vi "Begin.vi"() -> (0 "error out":errorcluster)   [LabVIEW 2013]
doc: "Called before other user functions, this VI is expected to open initial I/O refnums, load in file data, and do all program initialization. Notice that the <B>error out</B> terminal is simply used for data flow. Wiring it to other structures or subVIs ensures that this VI runs first."
uses:
  <vilib>/Rock Robotics/SystemInterfaces/DIO/FPGA_DIOPWMChannel.ctl
  <vilib>/Rock Robotics/WPI/SafetyOutput/WPI_SafetyOutputConfigMenu.ctl
  <vilib>/Rock Robotics/WPI/DriverStation/WPI_DriverStationRobotMode2.ctl
  <vilib>/Rock Robotics/WPI/Joystick/WPI_JoystickDeviceEnum.ctl
  <vilib>/Rock Robotics/SystemInterfaces/DIO/FPGA_DIORelayChannel.ctl
  <vilib>/Rock Robotics/SystemInterfaces/DIO/FPGA_DIOChannel.ctl
  <vilib>/Rock Robotics/SystemInterfaces/Typedef/FPGA_TypedefDigitalModule.ctl
  QueueAction.ctl
  <vilib>/Rock Robotics/WPI/Solenoid/WPI_SolenoidChannel.ctl
  TankDriveAction.ctl
  <vilib>/Rock Robotics/SystemInterfaces/Typedef/FPGA_TypedefSolenoidModule.ctl
  DoubleSolenoidAction.ctl
  RollerAction.ctl
  <vilib>/Rock Robotics/WPI/RobotDrive/WPI_RobotDriveOpen2MotorWithTalon.vi
  Robot Global Data.vi
  OutputErrors.vi
  <vilib>/Rock Robotics/WPI/Solenoid/WPI_SolenoidOpenSingle.vi
  <vilib>/Rock Robotics/WPI/Compressor/WPI_CompressorGetSetRefNum.vi
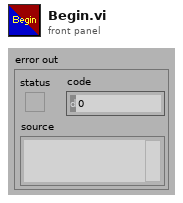
[diagram p1: front panel]
types:
  T1 = typedef "RollerAction.ctl" = enum16{"Init", "Off", "Forward", "Reverse"}
  T2 = typedef "FPGA_DIORelayChannel.ctl" = enum8{"Relay 1", "Relay 2", "Relay 3", "Relay 4", "Relay 5", "Relay 6", "Relay 7", "Relay 8", "Invalid"}
  T3 = typedef "FPGA_TypedefDigitalModule.ctl" = enum16{"Digital Module 1", "Digital Module 2"}
  T4 = typedef "DoubleSolenoidAction.ctl" = enum16{"Init", "Middle", "In", "Out"}
  T5 = typedef "WPI_SolenoidChannel.ctl" = enum8{"Solenoid 1", "Solenoid 2", "Solenoid 3", "Solenoid 4", "Solenoid 5", "Solenoid 6", "Solenoid 7", "Solenoid 8", "Invalid"}
  T6 = typedef "FPGA_TypedefSolenoidModule.ctl" = enum16{"Solenoid Module 1", "Solenoid Module 2"}
  T7 = typedef "QueueAction.ctl" = enum16{"Init", "SetValue", "Disable"}
  T8 = typedef "TankDriveAction.ctl" = enum16{"Init", "LinearDrive", "SetValue", "Disable"}
  T9 = typedef "WPI_JoystickDeviceEnum.ctl" = enum16{"USB 1", "USB 2", "USB 3", "USB 4", "Kinect 1", "Kinect 2"}
  T10 = typedef "FPGA_DIOChannel.ctl" = enum8{"DIO 1", "DIO 2", "DIO 3", "DIO 4", "DIO 5", "DIO 6", "DIO 7", "DIO 8", "DIO 9", "DIO 10", "DIO 11", "DIO 12", "DIO 13", "DIO 14", "Invalid"}
  T11 = typedef "WPI_DriverStationRobotMode2.ctl" = enum16{"Autonomous Disabled", "Autonomous Enabled", "Teleop Disabled", "Teleop Enabled", "Timeout", "Finish", "Test Disabled", "Test Enabled"}
  T12 = typedef "WPI_SafetyOutputConfigMenu.ctl" = enum16{"Enable", "Disable"}
  T13 = typedef "FPGA_DIOPWMChannel.ctl" = enum8{"PWM 1", "PWM 2", "PWM 3", "PWM 4", "PWM 5", "PWM 6", "PWM 7", "PWM 8", "PWM 9", "PWM 10", "Invalid"}
  T14 = typedef "WPI_JoystickDevRef.ctl" = cluster{"Device":T9}
  T15 = typedef "WPI_RobotDriveDevRef.ctl" = cluster{"DevStatus":errorcluster, "Motors[]":T16[], "Square Inputs":bool, "Max Output":dbl, "Isochronous":bool}
  T16 = typedef "WPI_MotorControlDeviceRef.ctl" = cluster{"DeviceStatus":errorcluster, "Type":enum16{"PWM", "CAN"}, "PWM":cluster{"Digital Module":T3, "PWM Channel":T13, "DeadBand":T17}, "CAN":cluster{"Device Number":u8, "Control Mode":T18, "Semaphore":T19, "Max Vout":dbl}, "Invert":bool, "TransformRef":T20, "InvTransformRef":T20}
  T17 = typedef "WPI_PWMDeadband.ctl" = cluster{"Name":string, "maxPositivePwm":i32, "minPositivePwm":i32, "centerPwm":i32, "maxNegativePwm":i32, "minNegativePwm":i32, "angularRange":u16}
  T18 = typedef "WPI_CANJaguar_ControlMode.ctl" = enum8{"Percent VBus", "Current", "Speed", "Position", "Voltage"}
  T19 = typedef "Semaphore RefNum" = refnum<k1>
  T20 = typedef "WPI_PWMTransform_ConPane.ctl" = refnum<vi>
  T21 = typedef "WPI_CompressorDevRef.ctl" = cluster{"DevStatus":errorcluster, "DigitalInputDevRef":T22, "RelayDevRef":T23}
  T22 = typedef "WPI_DigitalInputDevRef.ctl" = cluster{"DevStatus":errorcluster, "DIO Channel":T10, "Digital Module":T3}
  T23 = typedef "WPI_RelayDevRef.ctl" = cluster{"DevStatus":errorcluster, "Relay Channel":T2, "Digital Module":T3, "Relay Direction":T24}
  T24 = typedef "WPI_RelayDirection.ctl" = enum16{"Both directions", "Forward only", "Reverse only"}
  T25 = typedef "WPI_SolenoidDevRef.ctl" = cluster{"DevStatus":errorcluster, "Solenoid Module":T6, "Forward Solenoid Channel":T5, "Reverse Solenoid Channel":T5}
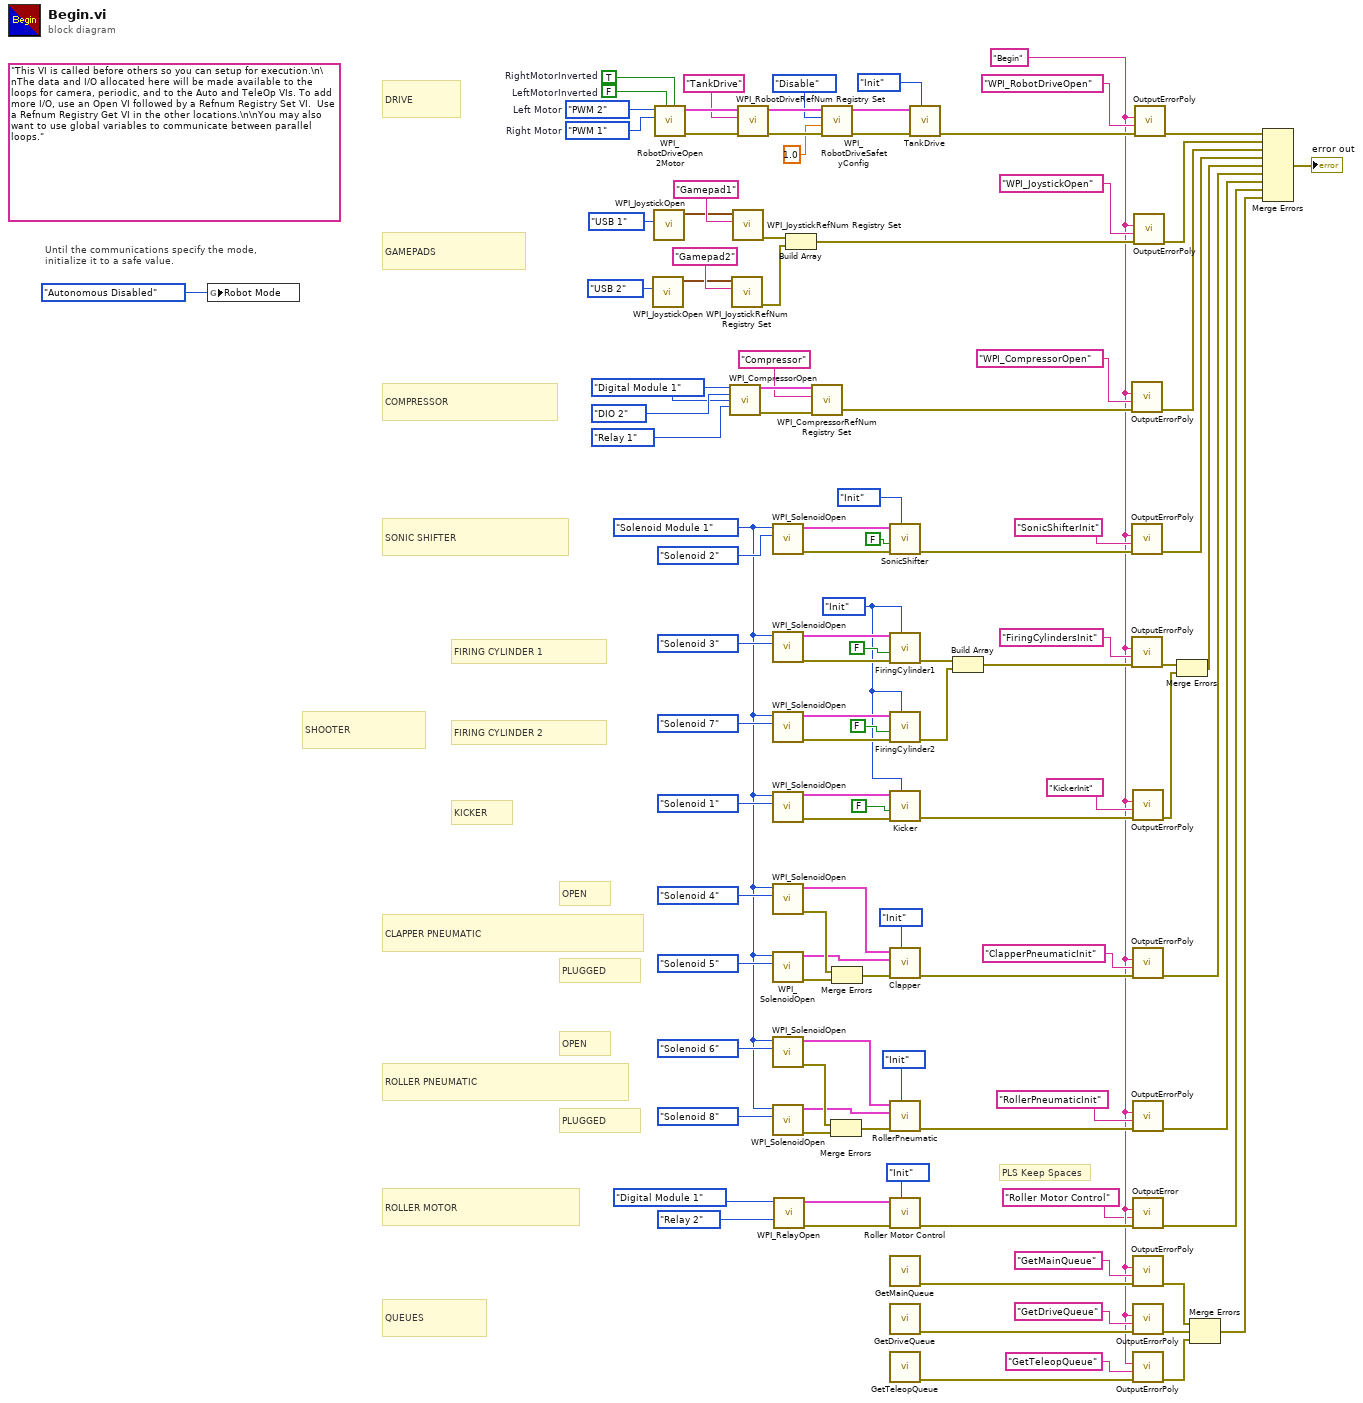
[diagram p0: block diagram]
diagram:
  w19 = FPGA_TypedefSolenoidModule."Solenoid Module 1" ("Solenoid Module (Module 1)")
  w42 = QueueAction."Init" ("Action")
  w88 = FPGA_TypedefDigitalModule."Digital Module 1" ("Pressure Switch\nand Relay Module")
  w2 = "Begin"
  (unwired) "This VI is called before others so you can setup for execution.\n\nThe data and I/O allocated here will be made available to the loops for camera, periodic, and to the Auto and TeleOp VIs. To add more I/O, use an Open VI followed by a Refnum Registry Set VI.  Use a Refnum Registry Get VI in the other locations.\n\nYou may also want to use global variables to communicate between parallel loops."
  w105 = FPGA_DIOPWMChannel."PWM 1"  # Right Motor
  w106 = FPGA_DIOPWMChannel."PWM 2"  # Left Motor
  w110 = FALSE  # LeftMotorInverted
  w111 = TRUE  # RightMotorInverted
  # "PLS Keep Spaces"
  # "ROLLER MOTOR"
  # "PLUGGED"
  # "OPEN"
  # "PLUGGED"
  # "OPEN"
  # "ROLLER PNEUMATIC"
  # "CLAPPER PNEUMATIC"
  # "SONIC SHIFTER"
  # "QUEUES"
  # "KICKER"
  # "FIRING CYLINDER 2"
  # "FIRING CYLINDER 1"
  # "SHOOTER"
  # "COMPRESSOR"
  # "GAMEPADS"
  # "DRIVE"
  # "Until the communications specify the mode,\ninitialize it to a safe value."
  n1 = global write "Robot Global Data.vi" "Robot Mode"(WPI_DriverStationRobotMode2."Autonomous Disabled" ("Robot Mode")) -> ()
  n2 = call <vilib>:"WPI_JoystickOpen.vi"("JoystickDevice"=WPI_JoystickDeviceEnum."USB 2") -> ("JoystickDevRef"=w84:T14)  [unwired: 10 in]
  n3 = call <vilib>:"WPI_JoystickOpen.vi"("JoystickDevice"=WPI_JoystickDeviceEnum."USB 1") -> ("JoystickDevRef"=w100:T14)  [unwired: 10 in]
  n4 = call-poly <vilib>:"WPI_RobotDriveOpen2Motor.vi"("Right Motor Inverted"=w111, "Left Motor Inverted"=w110, "Right Motor"=w105, "Left Motor"=w106) -> ("error out"=w107:errorcluster, "RobotDriveDevRef"=w109:T15)  [unwired: 1 in, 5 out]
  n5 = call <vilib>:"WPI_CompressorOpen.vi"("Pressure Switch Digital Module (Module 1)"=w88, "Pressure Switch DIO Channel"=FPGA_DIOChannel."DIO 2" ("Pressure Switch Channel"), "Relay Digital Module (Module 1)"=w88, "Relay Channel"=FPGA_DIORelayChannel."Relay 1") -> ("CompressorDevRef"=w92:T21, "error out"=w90:errorcluster)  [unwired: 1 in, 9 out]
  n6 = call <vilib>:"WPI_JoystickRefNum Registry Set.vi"("refnum name"="Gamepad2", "JoystickDevRef"=w84) -> ("error out"=w81:errorcluster)  [unwired: 8 in, 1 out]
  n7 = call <vilib>:"WPI_JoystickRefNum Registry Set.vi"("refnum name"="Gamepad1", "JoystickDevRef"=w100) -> ("error out"=w82:errorcluster)  [unwired: 8 in, 1 out]
  n8 = call <vilib>:"WPI_RobotDriveRefNum Registry Set.vi"("error in (no error)"=w107, "refnum name"="TankDrive", "RobotDriveDevRef"=w109) -> ("error out"=w98:errorcluster, "RobotDriveDevRef"=w104:T15)  [unwired: 7 out]
  n9 = call-poly <vilib>:"WPI_SolenoidOpen.vi"("Solenoid Channel"=WPI_SolenoidChannel."Solenoid 2", "Solenoid Module (Module 1)"=w19) -> ("error out"=w38:errorcluster, "SolenoidDevRef"=w39:T25)  [unwired: 8 in]
  n10 = call-poly <vilib>:"WPI_SolenoidOpen.vi"("Solenoid Channel"=WPI_SolenoidChannel."Solenoid 3", "Solenoid Module (Module 1)"=w19) -> ("error out"=w69:errorcluster, "SolenoidDevRef"=w72:T25)  [unwired: 8 in]
  n11 = call-poly <vilib>:"WPI_SolenoidOpen.vi"("Solenoid Channel"=WPI_SolenoidChannel."Solenoid 7", "Solenoid Module (Module 1)"=w19) -> ("error out"=w71:errorcluster, "SolenoidDevRef"=w68:T25)  [unwired: 8 in]
  n12 = call-poly <vilib>:"WPI_SolenoidOpen.vi"("Solenoid Channel"=WPI_SolenoidChannel."Solenoid 1", "Solenoid Module (Module 1)"=w19) -> ("error out"=w70:errorcluster, "SolenoidDevRef"=w67:T25)  [unwired: 8 in]
  n13 = call-poly <vilib>:"WPI_SolenoidOpen.vi"("Solenoid Channel"=WPI_SolenoidChannel."Solenoid 4", "Solenoid Module (Module 1)"=w19) -> ("error out"=w31:errorcluster, "SolenoidDevRef"=w29:T25)  [unwired: 8 in]
  n14 = call-poly <vilib>:"WPI_SolenoidOpen.vi"("Solenoid Channel"=WPI_SolenoidChannel."Solenoid 5", "Solenoid Module (Module 1)"=w19) -> ("error out"=w30:errorcluster, "SolenoidDevRef"=w27:T25)  [unwired: 8 in]
  n15 = call-poly <vilib>:"WPI_SolenoidOpen.vi"("Solenoid Channel"=WPI_SolenoidChannel."Solenoid 6", "Solenoid Module (Module 1)"=w19) -> ("error out"=w22:errorcluster, "SolenoidDevRef"=w17:T25)  [unwired: 8 in]
  n16 = call-poly <vilib>:"WPI_SolenoidOpen.vi"("Solenoid Channel"=WPI_SolenoidChannel."Solenoid 8", "Solenoid Module (Module 1)"=w19) -> ("error out"=w21:errorcluster, "SolenoidDevRef"=w16:T25)  [unwired: 8 in]
  n17 = call <vilib>:"WPI_RelayOpen.vi"("Relay Channel"=FPGA_DIORelayChannel."Relay 2", "Digital Module (Module 1)"=FPGA_TypedefDigitalModule."Digital Module 1") -> ("error out"=w5:errorcluster, "RelayDevRef"=w8:T23)  [unwired: 8 in]
  n18 = Build Array(w82, w81) -> (w80:errorcluster[])
  n19 = call <vilib>:"WPI_CompressorRefNum Registry Set.vi"("error in (no error)"=w90, "refnum name"="Compressor", "CompressorDevRef"=w92) -> ("error out"=w87:errorcluster)  [unwired: 7 in, 1 out]
  n20 = call <vilib>:"WPI_RobotDriveSafetyConfig.vi"("error in (no error)"=w98, "timeout (s)"=1.0, "mode"=WPI_SafetyOutputConfigMenu."Disable", "RobotDriveDevRef"=w104) -> ("error out"=w53:errorcluster, "RobotDriveDevRef"=w54:T15)  [unwired: 6 in]
  n21 = Merge Errors(w22, w21) -> (w18:errorcluster)
  n22 = Merge Errors(w31, w30) -> (w32:errorcluster)
  n23 = call "SonicShifter.vi"("Action"=QueueAction."Init", "error in (no error)"=w38, "Default Position"=FALSE, "SolenoidDevRef"=w39) -> ("error out"=w36:errorcluster)  [unwired: 7 in]
  n24 = call "FiringCylinder1.vi"("Action"=w42, "error in (no error)"=w69, "Default Position"=FALSE, "SolenoidDevRef"=w72) -> ("error out"=w74:errorcluster)  [unwired: 7 in]
  n25 = call "FiringCylinder2.vi"("Action"=w42, "error in (no error)"=w71, "Default Position"=FALSE, "SolenoidDevRef"=w68) -> ("error out"=w75:errorcluster)  [unwired: 7 in]
  n26 = call "Kicker.vi"("Action"=w42, "error in (no error)"=w70, "Default Position"=FALSE, "SolenoidDevRef"=w67) -> ("error out"=w76:errorcluster)  [unwired: 7 in]
  n27 = call "Clapper.vi"("State"=DoubleSolenoidAction."Init", "Error in"=w32, "Plugged"=w27, "Open"=w29) -> ("Error out"=w25:errorcluster)  [unwired: 7 in]
  n28 = call "RollerPneumatic.vi"("State"=DoubleSolenoidAction."Init", "Error in"=w18, "Plugged"=w16, "Open"=w17) -> ("Error out"=w15:errorcluster)  [unwired: 7 in]
  n29 = call "Roller Motor Control.vi"("Action"=RollerAction."Init", "Error in"=w5, "RelayDevRef"=w8) -> ("Error out"=w4:errorcluster)  [unwired: 8 in]
  n30 = call "GetMainQueue.vi"() -> ("error out"=w51:errorcluster)  [unwired: 10 in, 1 out]
  n31 = call "GetDriveQueue.vi"() -> ("error out"=w50:errorcluster)  [unwired: 10 in, 1 out]
  n32 = call "GetTeleopQueue.vi"() -> ("error out"=w49:errorcluster)  [unwired: 10 in, 1 out]
  n33 = call "TankDrive.vi"("DriveAction"=TankDriveAction."Init", "error in (no error)"=w53, "RobotDriveDevRef"=w54) -> ("error out"=w52:errorcluster)  [unwired: 8 in]
  n34 = Build Array(w74, w75) -> (w73:errorcluster[])
  n35 = call-poly "OutputErrorPoly.vi"("error in (no error)"=w87, "Causing VI"="WPI_CompressorOpen" ("Calling VI"), "Calling VI"=w2) -> ("error out"=w77:errorcluster)  [unwired: 8 in]
  n36 = call-poly "OutputErrorPoly.vi"("error in (no error)"=w36, "Causing VI"="SonicShifterInit", "Calling VI"=w2) -> ("error out"=w34:errorcluster)  [unwired: 8 in]
  n37 = call-poly "OutputErrorPoly.vi"("errors in"=w73, "Causing VI"="FiringCylindersInit", "Calling VI"=w2) -> ("error out"=w63:errorcluster)  [unwired: 8 in]
  n38 = call-poly "OutputErrorPoly.vi"("error in (no error)"=w76, "Causing VI"="KickerInit", "Calling VI"=w2) -> ("error out"=w62:errorcluster)  [unwired: 8 in]
  n39 = call-poly "OutputErrorPoly.vi"("error in (no error)"=w25, "Causing VI"="ClapperPneumaticInit", "Calling VI"=w2) -> ("error out"=w12:errorcluster)  [unwired: 8 in]
  n40 = call-poly "OutputErrorPoly.vi"("error in (no error)"=w15, "Causing VI"="RollerPneumaticInit", "Calling VI"=w2) -> ("error out"=w11:errorcluster)  [unwired: 8 in]
  n41 = call "OutputError.vi"("error in (no error)"=w4, "Causing VI"="Roller Motor Control", "Calling VI"=w2) -> ("error out"=w3:errorcluster)  [unwired: 8 in]
  n42 = call-poly "OutputErrorPoly.vi"("error in (no error)"=w51, "Causing VI"="GetMainQueue", "Calling VI"=w2) -> ("error out"=w46:errorcluster)  [unwired: 8 in]
  n43 = call-poly "OutputErrorPoly.vi"("error in (no error)"=w50, "Causing VI"="GetDriveQueue", "Calling VI"=w2) -> ("error out"=w47:errorcluster)  [unwired: 8 in]
  n44 = call-poly "OutputErrorPoly.vi"("error in (no error)"=w49, "Causing VI"="GetTeleopQueue", "Calling VI"=w2) -> ("error out"=w48:errorcluster)  [unwired: 8 in]
  n45 = call-poly "OutputErrorPoly.vi"("errors in"=w80, "Causing VI"="WPI_JoystickOpen", "Calling VI"=w2) -> ("error out"=w79:errorcluster)  [unwired: 8 in]
  n46 = call-poly "OutputErrorPoly.vi"("error in (no error)"=w52, "Causing VI"="WPI_RobotDriveOpen", "Calling VI"=w2) -> ("error out"=w78:errorcluster)  [unwired: 8 in]
  n47 = Merge Errors(w63, w62) -> (w61:errorcluster)
  n48 = Merge Errors(w46, w47, w48) -> (w6:errorcluster)
  n49 = Merge Errors(w78, w79, w77, w34, w61, w12, w11, w3, w6) -> (→"error out":errorcluster)
